vi "ParseVoltageInfo.vi"(5 "Input String":string="Clock1\tRG+\t-10.0\t+10.0\t2\t0\t0") -> (0 "Voltage":sgl format="%.1f", 1 "Name":string, 2 "Maximum":sgl format="%.2f", 3 "Minimum":sgl format="%.2f", 4 "Pin":string)   [LabVIEW 2014]
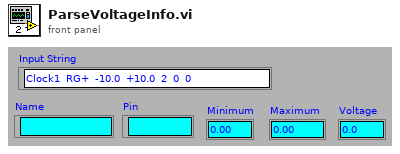
[diagram p1: front panel]
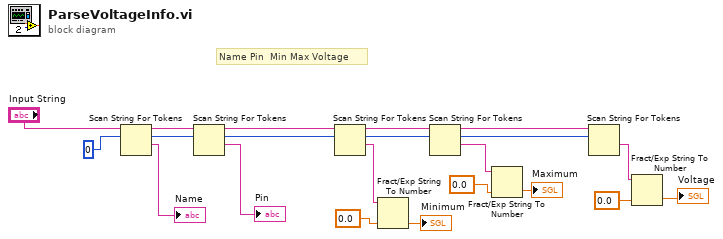
[diagram p0: block diagram]
diagram:
  # "Name Pin  Min Max Voltage"
  n1 = Scan String For Tokens(8:0 ("offset"), 9:"Input String") -> (1:→"Name":string, 2:w5:i32, 3:w6:string)  [unwired: 4 in, 1 out]
  n2 = Scan String For Tokens(8:w5, 9:w6) -> (1:→"Pin":string, 2:w3:i32, 3:w4:string)  [unwired: 4 in, 1 out]
  n3 = Scan String For Tokens(8:w3, 9:w4) -> (1:w21:string, 2:w19:i32, 3:w20:string)  [unwired: 4 in, 1 out]
  n4 = Fract/Exp String To Number(string=w21, default (0 dbl)=sgl 0.0 ("default (0L)")) -> (number=→"Minimum":sgl)  [unwired: 2 in, 1 out]
  n5 = Scan String For Tokens(8:w19, 9:w20) -> (1:w18:string, 2:w8:i32, 3:w9:string)  [unwired: 4 in, 1 out]
  n6 = Fract/Exp String To Number(string=w18, default (0 dbl)=sgl 0.0 ("default (0L)")) -> (number=→"Maximum":sgl)  [unwired: 2 in, 1 out]
  n7 = Scan String For Tokens(8:w8, 9:w9) -> (1:w15:string)  [unwired: 4 in, 3 out]
  n8 = Fract/Exp String To Number(string=w15, default (0 dbl)=sgl 0.0) -> (number=→"Voltage":sgl)  [unwired: 2 in, 1 out]
